vi "AD5781SetVolt.vi"(3 "Send":bool=TRUE, 5 "SetVolt":u32 format="%032b") -> (0 "Readback":u32 format="%024b", 1 "Readback 0":u32 format="%032b", 2 "timedOut":bool)   [LabVIEW 2014]
uses:
  <vilib>/rvi/Emulation/niFpgaGetClockAttributes.vi
  <vilib>/rvi/Emulation/niFpgaSctlEmulationGetInTimedLoop.vi
  <vilib>/rvi/Emulation/niFpgaEmulationReportErrorSimple.vi
  <vilib>/rvi/eio/common/nirviEmuTemplateMethod_errors.vi
  <vilib>/rvi/Emulation/niFpgaCriticalErrorInLSC.vi
  Code/FPGA SPI_Globals.vi
  <vilib>/rvi/Emulation/niFpgaProcessEmulError.vi
  <vilib>/eio/EIONode/EIONode.xnode
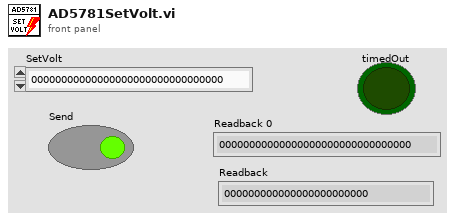
[diagram p1: front panel]
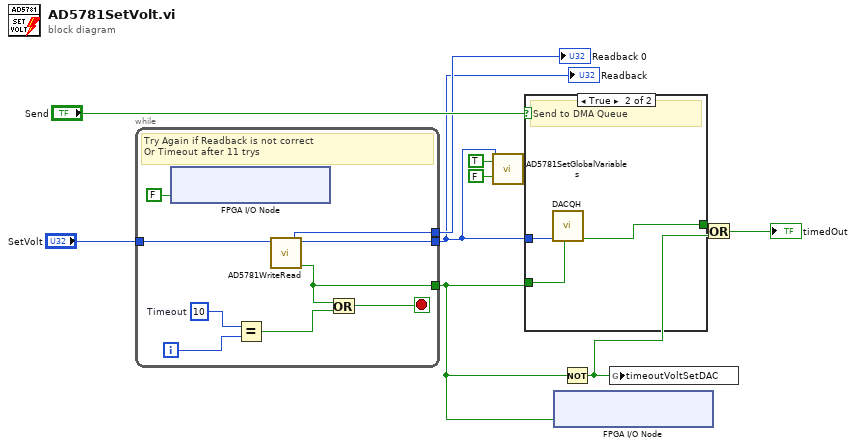
[diagram p0: block diagram]
diagram:
  n1 = while {
    tunnel: "SetVolt" -> [w19]
    tunnel: [w14] -> w3
    tunnel: [w13] -> w8
    tunnel: [w11] -> w7
    i -> [w18]
    stop <- w16 stop-if-true
    w17 = 10  # Timeout
    # "Try Again if Readback is not correct\nOr Timeout after 11 trys"
    n2 = xnode "FPGA I/O Node"("voltSetFlagDio10Con1"=FALSE) -> ()  [unwired: 1 in, 1 out]
    n3 = Equal?(x=w17, y=w18) -> (x = y?=w15:bool)
    n4 = call "AD5781WriteRead.vi"("Write"=w19) -> ("WriteEqualsRead"=w13:bool, "Readback 0"=w11:u32, "Readback"=w14:u32)  [unwired: 5 in]
    n5 = Or(x=w13, y=w15) -> (x .or. y?=w16:bool)
  }
  "Readback" <- w3
  "Readback 0" <- w7
  n6 = call "AD5781SetGlobalVariables.vi"("actDACRegister"=w3, "write actDACRegister"=TRUE, "write setDACRegister"=FALSE) -> ()  [unwired: 17 in]
  n7 = case shown="True" "Send" {
    tunnel: w3 -> [_ w20]
    tunnel: w8 -> [_ w22]
    tunnel: [_ w21] -> w4
    frame False {
    }
    frame True {
      # "Send to DMA Queue"
      n8 = call "DACQH.vi"("writeEqualsRead?"=w22, "Readback"=w20) -> ("DACQuWriteTimeout"=w21:bool)  [unwired: 9 in]
    }
  }
  n9 = xnode "FPGA I/O Node"("voltSetFlagDio10Con1"=w8) -> ()  [unwired: 1 in, 1 out]
  n10 = Not(x=w8) -> (.not. x?=w6:bool)
  n11 = global write "FPGA SPI_Globals.vi" "timeoutVoltSetDAC"(w6) -> ()
  n12 = Or(x=w4, y=w6) -> (x .or. y?=→"timedOut":bool)
